vi "Method.vi"(4 "Value":refnum<class "Abs_Numeric.lvclass">) -> (1 "Result":refnum<class "ConvertTo_U8.lvclass">)   [LabVIEW 2021, in "ConvertTo_U8.lvclass"]
uses:
  ConvertTo_U8.lvclass
  Abs_Types/Numeric/Abs_Numeric.lvclass
  ConvertTo_U8.lvclass/ConvertTo_U8.ctl
  Properties/Write Value.vi
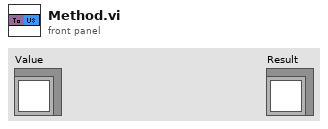
[diagram p1: front panel]
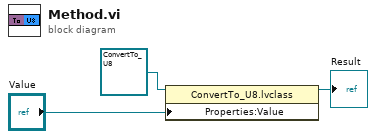
[diagram p0: block diagram]
diagram:
  n1 = property class="ConvertTo_U8.lvclass"(reference=refnum<class "ConvertTo_U8.lvclass"> refnum ("ConvertTo_DBL.lvclass"), "Properties:Value"="Value") -> (reference out=→"Result":refnum<class "ConvertTo_U8.lvclass">)  [unwired: 1 in, 1 out]
